vi "NXT_MIDBRAIN REVERSE.vi"(2 "_sensorData":T2={"_irData"={"_irDistance"=0, "_irHeading"=0, "_irTimestamp"=0}, "_batteryVoltage"=0, "_NXTButtonStates"=[FALSE, FALSE, FALSE]}, 3 "Behavior #":i32, 4 "Previous Motor Position":T1={"_rudderCommand"=7, "_propCommand"=7, "_irServoCommand"=7}, 5 "Behavior Weights":T4=[0, 0, 0, 0, 0, 0]) -> (0 "Rudder Command":i32, 1 "Behavior Output":T5)   [LabVIEW 2012]
uses:
  behaviorOutput_t.ctl
  behaviorWeights_t.ctl
  sensorData_t.ctl
  irData_t.ctl
  motorCommands_t.ctl
panel:
  in  "greater250":i32
  in  "Goodness":i32=50
  in  "lessthat100":i32
  in  "between150_100":i32
  in  "between200_150":i32
  in  "between250_200":i32
  in  "Speed":i32=1
  # "DEBUG"
  # "L\nE\nF\nT"
  # "C\nE\nN\nT\nE\nR"
  # "R\nI\nG\nH\nT"
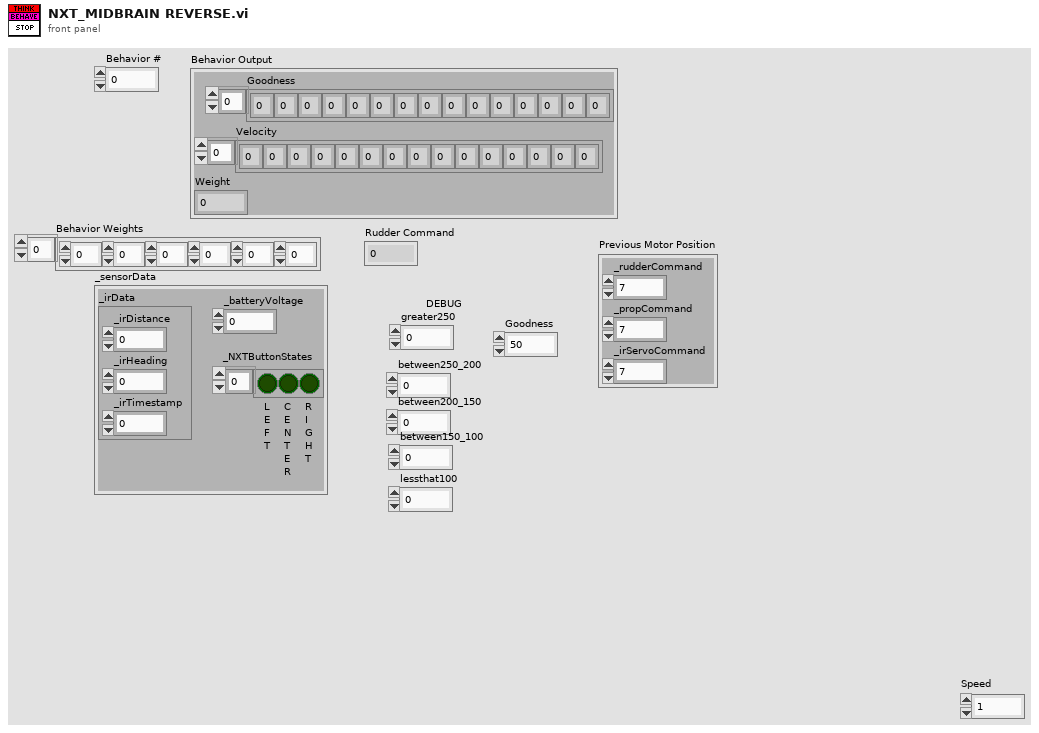
[diagram p1: front panel]
types:
  T1 = typedef "motorCommands_t.ctl" = cluster{"_rudderCommand":i8, "_propCommand":i8, "_irServoCommand":i8}
  T2 = typedef "sensorData_t.ctl" = cluster{"_irData":T3, "_batteryVoltage":i32, "_NXTButtonStates":bool[]}
  T3 = typedef "irData_t.ctl" = cluster{"_irDistance":i32, "_irHeading":i32, "_irTimestamp":u32}
  T4 = typedef "behaviorWeights_t.ctl" = i8[]
  T5 = typedef "behaviorOutput_t.ctl" = cluster{"Goodness":i8[], "Velocity":i8[], "Weight":i8}
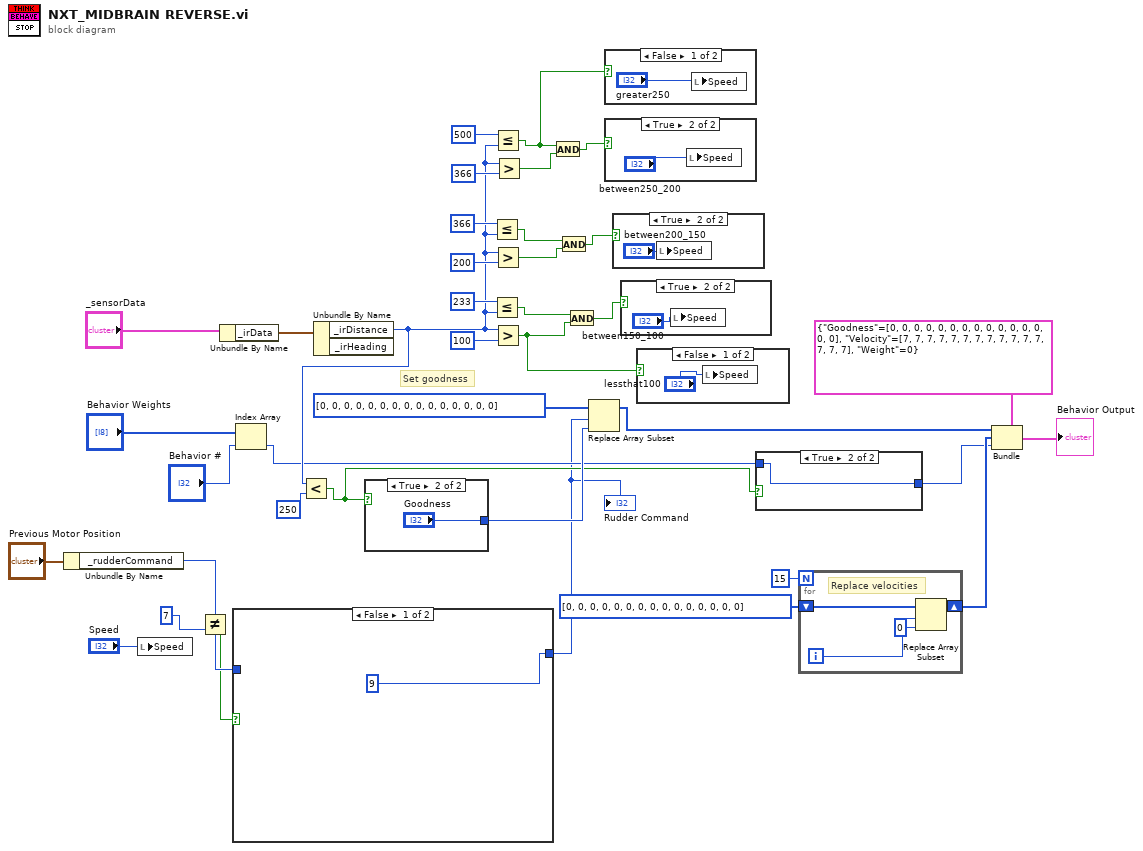
[diagram p0: block diagram]
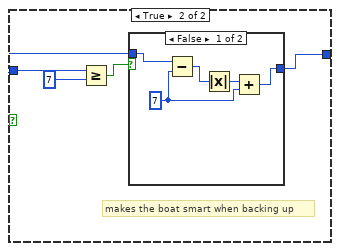
[diagram p2: hidden frame]
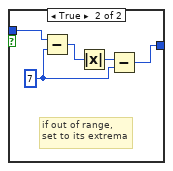
[diagram p3: hidden frame]
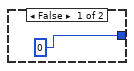
[diagram p4: hidden frame]
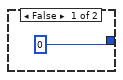
[diagram p5: hidden frame]
diagram:
  # "Set goodness"
  n1 = Unbundle By Name("Previous Motor Position") -> ("_rudderCommand"=w3:i8)
  n2 = local write "Speed"("Speed") -> ()
  n3 = Not Equal?(x=w3, y=7) -> (x != y?=w2:bool)
  n4 = Unbundle By Name("_sensorData") -> ("_irData"=w33:T3)
  n5 = case shown="False" w2 {
    tunnel: w3 -> [_ w41]
    tunnel: [9 w40] -> w4
    frame False {
    }
    frame True {
      # "makes the boat smart when backing up"
      n6 = Greater Or Equal?(x=w41, y=7) -> (x >= y?=w42:bool)
      n7 = case shown="False" w42 {
        tunnel: w41 -> [w45 w53]
        tunnel: [w44 w49] -> w40
        frame False {
          w47 = 7
          n8 = Subtract(x=w45, y=w47) -> (x-y=w46:i32)
          n9 = Absolute Value(x=w46) -> (abs(x)=w48:i32)
          n10 = Add(x=w48, y=w47) -> (x+y=w44:i32)
        }
        frame True {
          w51 = 7
          # "if out of range,\nset to its extrema"
          n11 = Subtract(x=w53, y=w51) -> (x-y=w52:i32)
          n12 = Absolute Value(x=w52) -> (abs(x)=w50:i32)
          n13 = Subtract(x=w50, y=w51) -> (x-y=w49:i32)
        }
      }
    }
  }
  "Rudder Command" <- w4
  n14 = Index Array(array="Behavior Weights", index="Behavior #") -> (element=w6:i8)
  n15 = Unbundle By Name(w33) -> ("_irDistance"=w8:i32)  [unwired: 1 out]
  n16 = Less?(x=w8, y=250) -> (x < y?=w7:bool)
  n17 = case shown="True" w7 {
    tunnel: [0 ("Numeric 2") "Goodness"] -> w12
    frame False {
    }
    frame True {
    }
  }
  n18 = Less Or Equal?(x=366 ("y"), y=w8) -> (x <= y?=w21:bool)
  n19 = Less Or Equal?(x=233 ("y"), y=w8) -> (x <= y?=w19:bool)
  n20 = Less Or Equal?(x=500 ("y"), y=w8) -> (x <= y?=w17:bool)
  n21 = Greater?(x=w8, y=200) -> (0:w20:bool)
  n22 = Greater?(x=w8, y=100) -> (0:w13:bool)
  n23 = Greater?(x=w8, y=366) -> (0:w22:bool)
  n24 = And(x=w17, y=w22) -> (x .and. y?=w18:bool)
  n25 = And(x=w21, y=w20) -> (x .and. y?=w16:bool)
  n26 = And(x=w19, y=w13) -> (x .and. y?=w15:bool)
  n27 = Replace Array Subset(array=i8[] [0, 0, 0, 0, 0, 0, 0, 0, 0, 0, 0, 0, 0, 0, 0] ("Goodness"), new element=w12, index=w4) -> (w30:i8[])
  n28 = case shown="False" w17 {
    frame False {
      n29 = local write "Speed"("greater250") -> ()
    }
    frame True {
    }
  }
  n30 = case shown="True" w18 {
    frame False {
    }
    frame True {
      n31 = local write "Speed"("between250_200") -> ()
    }
  }
  n32 = case shown="True" w16 {
    frame False {
    }
    frame True {
      n33 = local write "Speed"("between200_150") -> ()
    }
  }
  n34 = case shown="True" w15 {
    frame False {
    }
    frame True {
      n35 = local write "Speed"("between150_100") -> ()
    }
  }
  n36 = case shown="False" w13 {
    frame False {
      n37 = local write "Speed"("lessthat100") -> ()
    }
    frame True {
    }
  }
  n38 = case shown="True" w7 {
    tunnel: w6 -> [_ w62]
    tunnel: [0 w62] -> w5
    frame False {
    }
    frame True {
    }
  }
  n39 = for {
    N: 15 -> [_]
    shift-right: [w66] -> w29
    shift-left: i8[] [0, 0, 0, 0, 0, 0, 0, 0, 0, 0, 0, 0, 0, 0, 0] ("Goodness") -> [w64]
    i -> [w63]
    # "Replace velocities"
    n40 = Replace Array Subset(array=w64, new element=i8 0 ("new element/subarray"), index=w63) -> (w66:i8[])
  }
  n41 = Bundle(cluster=T5 {"Goodness"=[0, 0, 0, 0, 0, 0, 0, 0, 0, 0, 0, 0, 0, 0, 0], "Velocity"=[7, 7, 7, 7, 7, 7, 7, 7, 7, 7, 7, 7, 7, 7, 7], "Weight"=0} ("Behavior Output"), "Goodness"=w30, "Velocity"=w29, "Weight"=w5) -> (→"Behavior Output":T5)
